vi "Put_Down_Card.vi"(7 "error in":errorcluster, 10 "VISA Refnum in":refnum<visa-resource-name>="COM3") -> (0 "error out":errorcluster, 3 "Machine Out":refnum<visa-resource-name>)   [LabVIEW 2018]
doc: "Example interface for controlling uArm Swift Pro."
panel:
  in  "Write Buffer":string="G90 G0 X1\n"
  out "read buffer":string
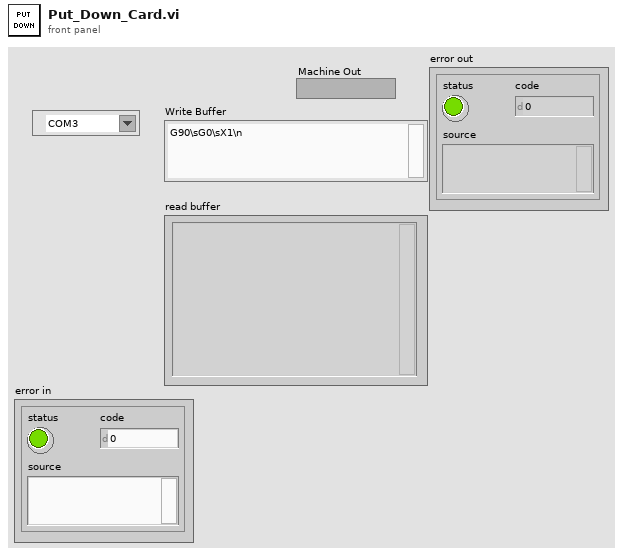
[diagram p1: front panel]
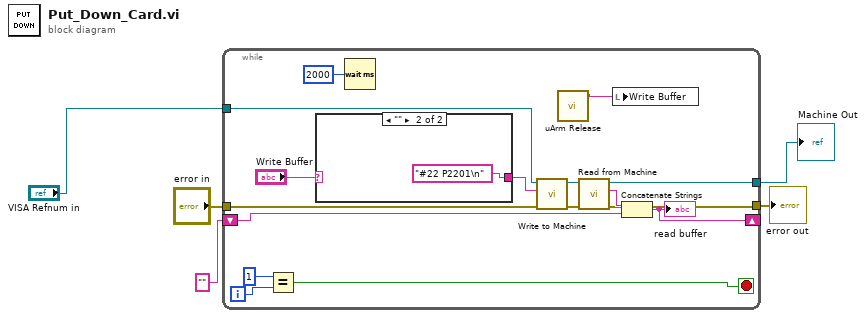
[diagram p0: block diagram]
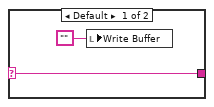
[diagram p2: hidden frame]
diagram:
  n1 = while {
    tunnel: "VISA Refnum in" -> [w19]
    tunnel: "error in" -> [w16]
    shift-right: [w17] -> _
    shift-left: "" -> [w18]
    tunnel: [w15] -> w2
    tunnel: [w10] -> w1
    i -> [w9]
    stop <- w7 stop-if-true
    n2 = Equal?(x=1, y=w9) -> (x = y?=w7:bool)
    n3 = case shown="\"\"" "Write Buffer" {
      selector: "Write Buffer" -> [w23 _]
      tunnel: [w23 "#22 P2201\n"] -> w20
      frame Default {
        n4 = local write "Write Buffer"("") -> ()
      }
      frame "" {
      }
    }
    n5 = Wait (ms)(milliseconds to wait=u32 2000) -> ()  [unwired: 1 out]
    n6 = call "Write to Machine .vi"("error in (no error)"=w16, "G-Code String In"=w20, "Machine In"=w19) -> ("error out"=w13:errorcluster, "Machine Out"=w12:refnum<visa-resource-name>)  [unwired: 7 in]
    n7 = call "uArm Release.vi"() -> ("G-Code String"=w11:string)  [unwired: 11 in]
    n8 = call "Read from Machine.vi"("error in (no error)"=w13, "Machine In"=w12) -> ("error out"=w10:errorcluster, "read buffer"=w14:string, "Machine Out"=w15:refnum<visa-resource-name>)  [unwired: 7 in]
    n9 = local write "Write Buffer"(w11) -> ()
    n10 = Concatenate Strings(w14, w18) -> (w17:string)
    "read buffer" <- w17
  }
  "Machine Out" <- w2
  "error out" <- w1
